vi "OS Simulator - V3.vi"() -> ()   [LabVIEW 2020]
uses:
  <vilib>/numeric/Random Number (Range) U64.vi
  <vilib>/numeric/Random Number (Range) DBL.vi
  <vilib>/numeric/Random Number (Range) I64.vi
  <vilib>/numeric/sub_Random U32.vi
panel:
  out "number":u64
  in  "Probabilidad de Memoria":dbl(slide)=15.0 min=0.0 max=80.0 step=1.0 scale=0.0..100.0
  in  "Numeric 4":dbl
  in  "Tamaño de Páginas":dbl(slide)=8.0 min=0.0 max=64.0 step=4.0 scale=4.0..64.0
  in  "Tamaño de Ram":dbl(slide)=64.0 min=0.0 max=80.0 step=4.0 scale=32.0..256.0
  in  "MEMORY MAP":string[](array[string])
  in  "TAP":string[][](table)
  in  "USING DISK":string
  in  "DISK WAITING":string[](array[string])
  in  "PROCESOS":dbl=20.0
  in  "VELOCIDAD":dbl(slide)=1000.0 min=0.0 max=2000.0 step=500.0
  in  "String":string
  in  "NEW":string[](array[string])
  in  "Numeric":dbl
  in  "FINISHED":string[](array[string])
  in  "PRINT":string
  in  "I/O WAITING":string[](array[string])
  in  "TABLA DE SALIDA":string[][](table)
  in  "RUNNING":string
  in  "READY":string[](array[string])
  in  "PROGRAM CONTROL BLOCK":string[][](table)
  in  "Tiempo Prom de Impresión":dbl(slide)=15.0 min=0.0 max=80.0 step=1.0 scale=10.0..80.0
  in  "Probabilidad de Impresión":dbl(slide)=50.0 min=0.0 max=100.0 step=1.0 scale=0.0..100.0
  in  "Duración Media de un Proceso":dbl(slide)=15.0 min=0.0 max=100.0 step=1.0 scale=0.0..100.0
  in  "Probabilidad de Proceso":dbl(slide) min=0.0 max=100.0 step=1.0 scale=0.0..100.0
  in  "Quantum":dbl(slide)=5.0 min=0.0 max=20.0 step=1.0 scale=0.0..20.0
  out "Play":bool
  out "Pause":bool
  in  "Play / Pause":bool=TRUE
  out "CLOCK":i32
  in  "Stop":bool
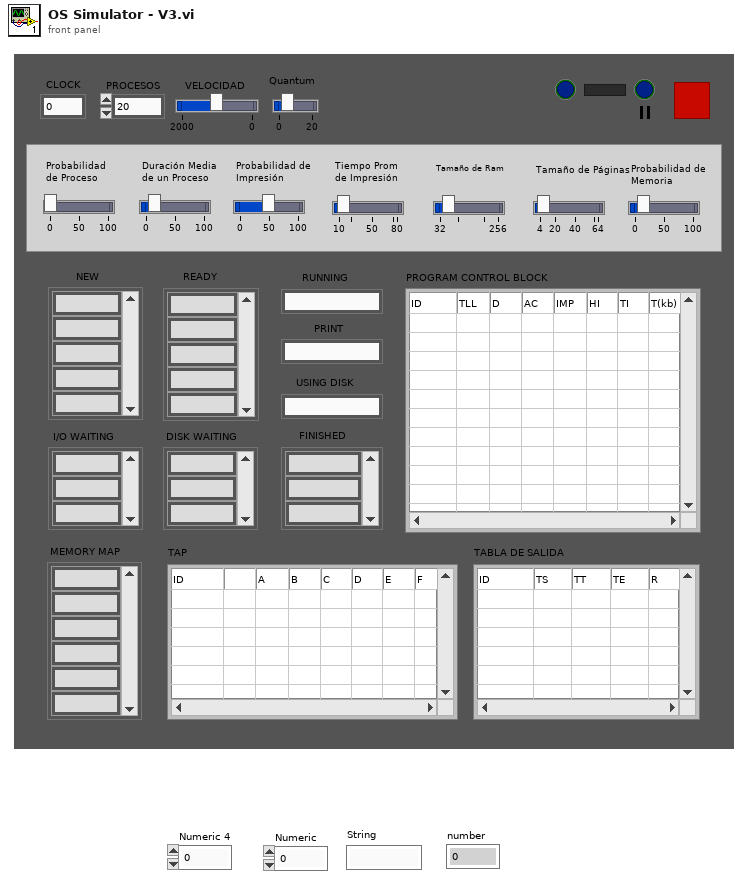
[diagram p1: front panel]
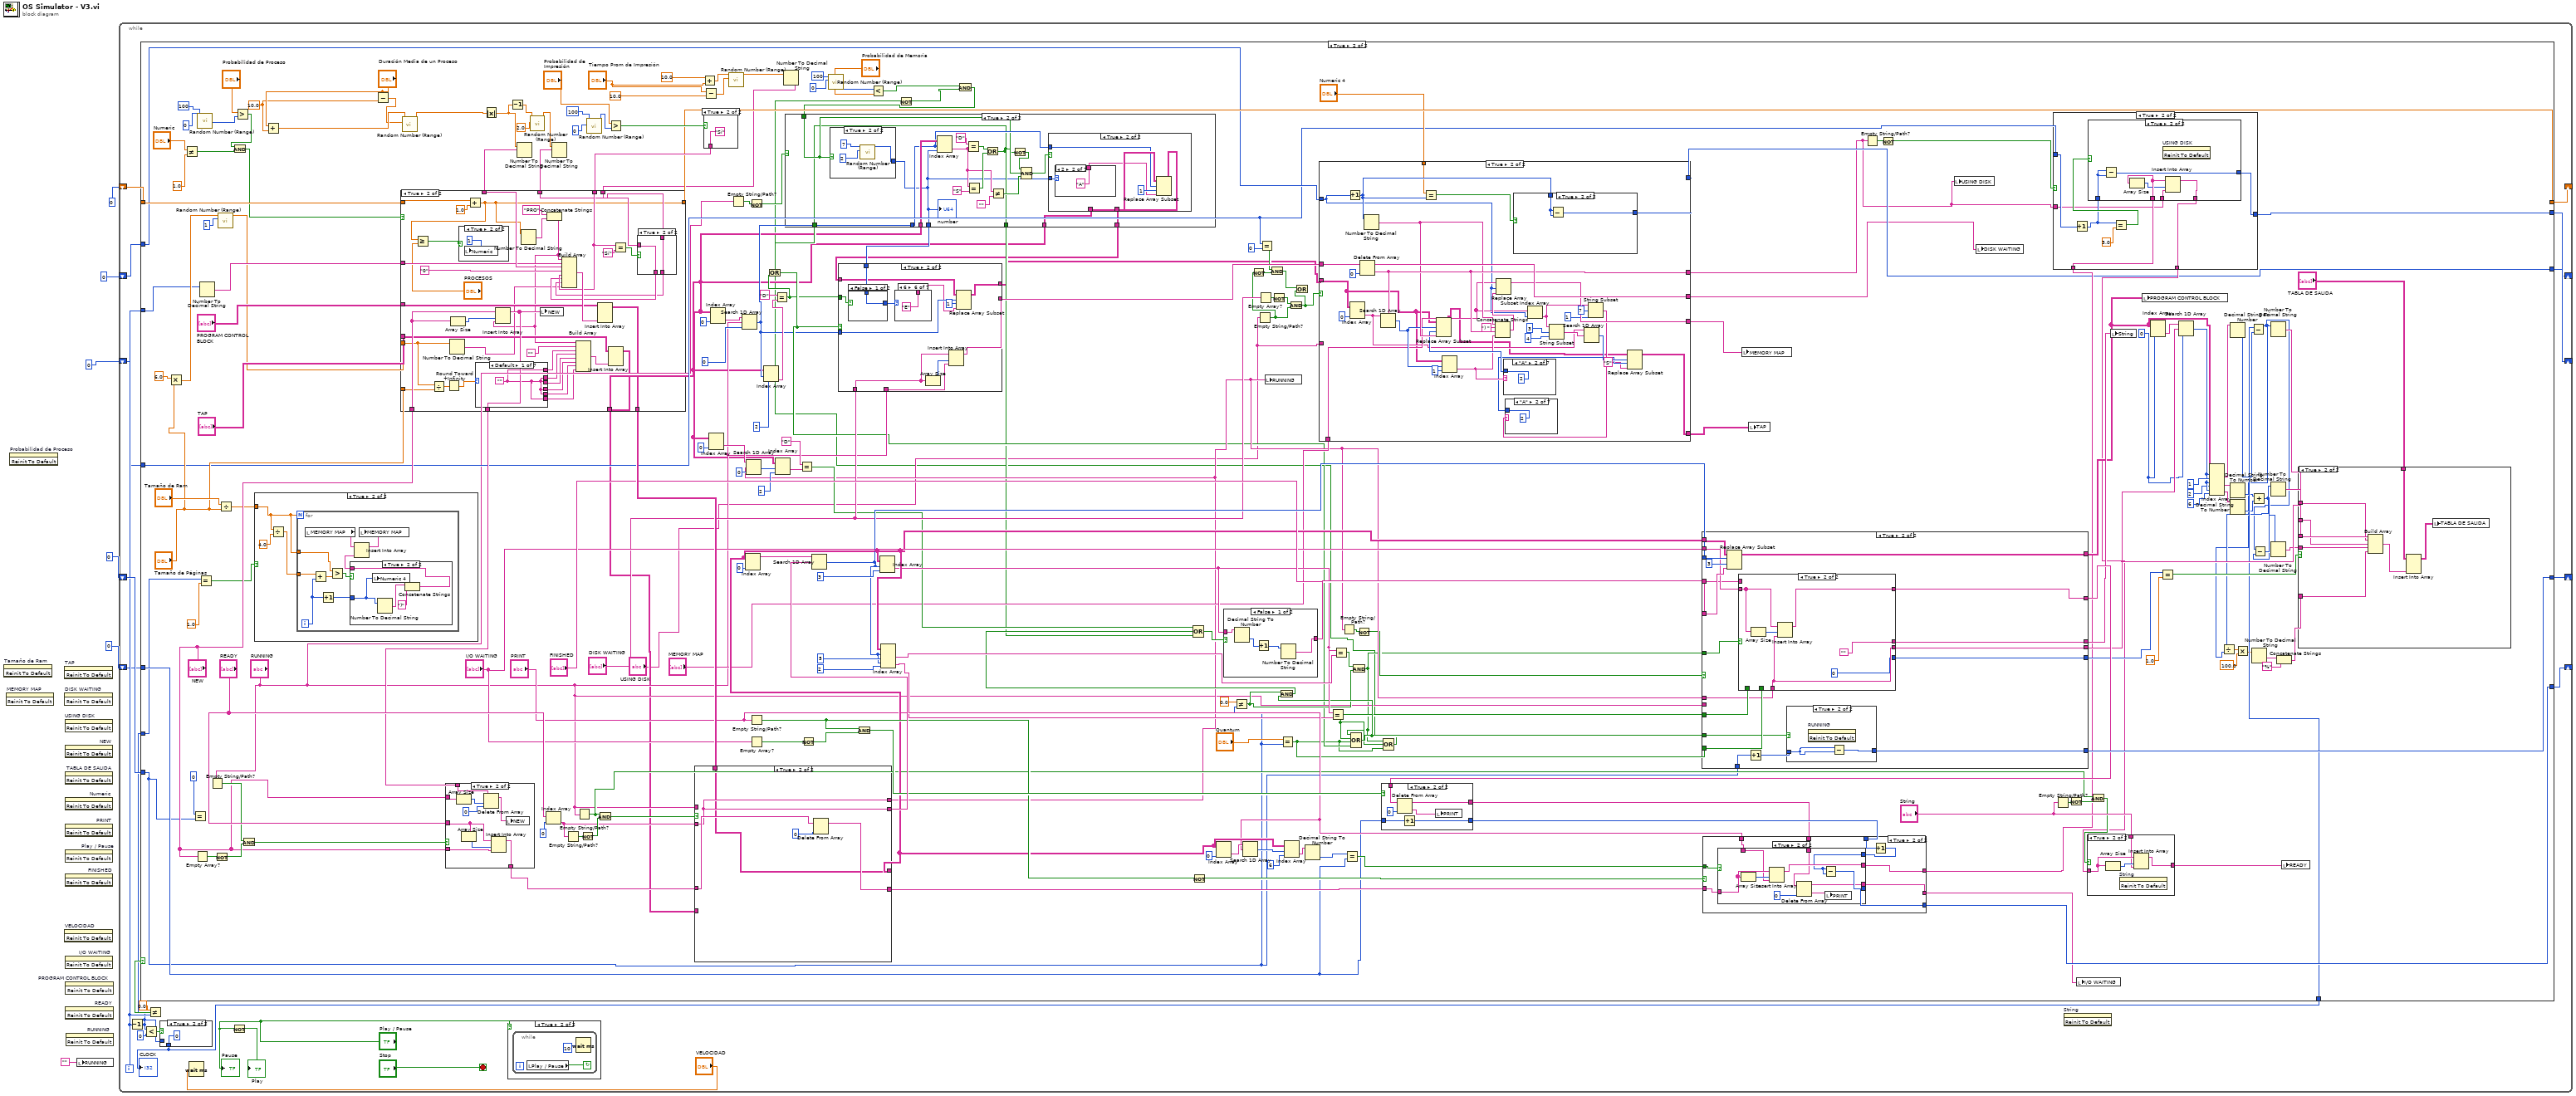
[diagram p0: block diagram]
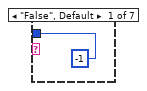
[diagram p5: hidden frame]
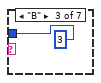
[diagram p6: hidden frame]
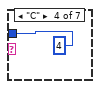
[diagram p7: hidden frame]
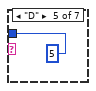
[diagram p8: hidden frame]
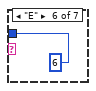
[diagram p9: hidden frame]
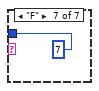
[diagram p10: hidden frame]
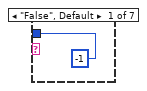
[diagram p11: hidden frame]
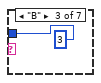
[diagram p12: hidden frame]
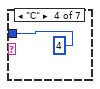
[diagram p13: hidden frame]
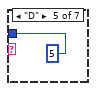
[diagram p14: hidden frame]
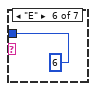
[diagram p15: hidden frame]
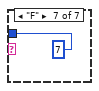
[diagram p16: hidden frame]
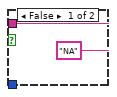
[diagram p19: hidden frame]
diagram:
  n1 = invoke on="Tamaño de Ram" class="Slide (strict)" method="Reinit To Default"() -> ()  [unwired: 3 in, 3 out]
  n2 = invoke on="MEMORY MAP" class="Arr (strict)" method="Reinit To Default"() -> ()  [unwired: 3 in, 3 out]
  n3 = invoke on="Probabilidad de Proceso" class="Slide (strict)" method="Reinit To Default"() -> ()  [unwired: 3 in, 3 out]
  n4 = invoke on="TAP" class="Tbl (strict)" method="Reinit To Default"() -> ()  [unwired: 3 in, 3 out]
  n5 = invoke on="DISK WAITING" class="Arr (strict)" method="Reinit To Default"() -> ()  [unwired: 3 in, 3 out]
  n6 = invoke on="VELOCIDAD" class="Slide (strict)" method="Reinit To Default"() -> ()  [unwired: 3 in, 3 out]
  n7 = invoke on="USING DISK" class="Str" method="Reinit To Default"() -> ()  [unwired: 3 in, 3 out]
  n8 = invoke on="NEW" class="Arr (strict)" method="Reinit To Default"() -> ()  [unwired: 3 in, 3 out]
  n9 = invoke on="TABLA DE SALIDA" class="Tbl (strict)" method="Reinit To Default"() -> ()  [unwired: 3 in, 3 out]
  n10 = invoke on="Numeric" class="DigNum (strict)" method="Reinit To Default"() -> ()  [unwired: 3 in, 3 out]
  n11 = invoke on="PRINT" class="Str" method="Reinit To Default"() -> ()  [unwired: 3 in, 3 out]
  n12 = invoke on="Play / Pause" class="Bool (strict)" method="Reinit To Default"() -> ()  [unwired: 3 in, 3 out]
  n13 = invoke on="FINISHED" class="Arr (strict)" method="Reinit To Default"() -> ()  [unwired: 3 in, 3 out]
  n14 = invoke on="I/O WAITING" class="Arr (strict)" method="Reinit To Default"() -> ()  [unwired: 3 in, 3 out]
  n15 = invoke on="PROGRAM CONTROL BLOCK" class="Tbl (strict)" method="Reinit To Default"() -> ()  [unwired: 3 in, 3 out]
  n16 = invoke on="READY" class="Arr (strict)" method="Reinit To Default"() -> ()  [unwired: 3 in, 3 out]
  n17 = invoke on="RUNNING" class="Str" method="Reinit To Default"() -> ()  [unwired: 3 in, 3 out]
  n18 = local write "RUNNING"("") -> ()
  n19 = while {
    shift-right: [w24] -> _
    shift-left: 0 -> [w23]
    shift-right: [w19] -> _
    shift-left: 0 -> [w20]
    shift-right: [w14] -> _
    shift-left: 0 -> [w15]
    shift-right: [w9] -> _
    shift-left: 0 -> [w10]
    shift-right: [w7] -> _
    shift-left: 0 -> [w8]
    i -> [w18]
    stop <- "Stop" stop-if-true
    n20 = Decrement(x=w18) -> (x-1=w11:i32)
    n21 = Less?(x=w11, y=0) -> (x < y?=w17:bool)
    n22 = Not Equal?(x=0.0, y=w18) -> (x != y?=w22:bool)
    n23 = case shown="True" w17 {
      tunnel: [w28 0] -> w13
      tunnel: w11 -> [w28 _]
      frame False {
      }
      frame True {
      }
    }
    "CLOCK" <- w13
    n24 = case shown="True" w22 {
      tunnel: [w34 w225] -> w24
      tunnel: w23 -> [w34 w224]
      tunnel: w18 -> [_ w113]
      tunnel: w20 -> [w33 w94]
      tunnel: [w33 w189] -> w19
      tunnel: w15 -> [w32 w168]
      tunnel: [w32 w178] -> w14
      tunnel: w13 -> [_ w142]
      tunnel: w11 -> [_ w110]
      tunnel: w10 -> [w31 w68]
      tunnel: [w31 w77] -> w9
      tunnel: w8 -> [w30 w74]
      tunnel: [w30 w73] -> w7
      frame False {
      }
      frame True {
        w130 = 0 ("disabled index (col)")
        w228 = 10.0 ("y")
        n25 = Multiply(x=6.0, y="Tamaño de Páginas") -> (x*y=w116:dbl)
        n26 = Not Equal?(x="Numeric", y=1.0) -> (x != y?=w210:bool)
        n27 = Equal?(x=0, y=w94) -> ()  [unwired: 1 out]
        n28 = Empty Array?(array="NEW") -> (empty?=w207:bool)
        n29 = call-poly <vilib>:"Random Number (Range).vi"("lower bound (-100)"=0, "upper bound (100)"=100) -> ("number"=w204:i64)  [unwired: 9 in]
        n30 = Equal?(x=w110, y=1.0) -> (x = y?=w112:bool)
        n31 = Number To Decimal String(number=w113) -> (decimal integer string=w237:string)  [unwired: 1 in]
        n32 = Empty String/Path?(string/path="RUNNING") -> (empty?=w200:bool)
        n33 = Not(x=w207) -> (.not. x?=w206:bool)
        n34 = call-poly <vilib>:"Random Number (Range).vi"("lower bound (0)"=1, "upper bound (100)"=w116) -> ("number"=w119:dbl)  [unwired: 9 in]
        n35 = Divide(x="Tamaño de Ram", y="Tamaño de Páginas") -> (x/y=w111:dbl)
        n36 = Greater?(x="Probabilidad de Proceso", y=w204) -> (0:w211:bool)
        n37 = And(x=w211, y=w210) -> (x .and. y?=w209:bool)
        n38 = And(x=w200, y=w206) -> (x .and. y?=w187:bool)
        n39 = case shown="True" w112 {
          tunnel: w111 -> [_ w300]
          frame False {
          }
          frame True {
            n40 = Divide(x=w300, y=4.0) -> (x/y=w301:dbl)
            n41 = for {
              N: w300 -> [_]
              tunnel: w301 -> [w309]
              tunnel: w300 -> [w306]
              i -> [w303]
              n42 = local read "MEMORY MAP"() -> (w310:string[])
              n43 = Add(x=w309, y=w303) -> (x+y=w305:dbl)
              n44 = Increment(x=w303) -> (x+1=w304:i32)
              n45 = Greater?(x=w306, y=w305) -> (0:w307:bool)
              n46 = case shown="True" w307 {
                tunnel: ["NA" w314] -> w308
                tunnel: w304 -> [_ w313]
                frame False {
                }
                frame True {
                  n47 = local write "Numeric 4"(w313) -> ()
                  n48 = Number To Decimal String(number=w313) -> (decimal integer string=w316:string)  [unwired: 1 in]
                  n49 = Concatenate Strings(w316, ")" ("string")) -> (w314:string)
                }
              }
              n50 = Insert Into Array(array=w310, new element=w308) -> (w311:string[])  [unwired: 1 in]
              n51 = local write "MEMORY MAP"(w311) -> ()
            }
          }
        }
        n52 = Add(x="Duración Media de un Proceso", y=w228) -> (x+y=w235:dbl)
        n53 = Subtract(x="Duración Media de un Proceso", y=w228) -> (x-y=w233:dbl)
        n54 = call-poly <vilib>:"Random Number (Range).vi"("lower bound (0)"=w233, "upper bound (100)"=w235) -> ("number"=w157:dbl)  [unwired: 9 in]
        n55 = Absolute Value(x=w157) -> (abs(x)=w156:dbl)
        n56 = Decrement(x=w156) -> (x-1=w216:dbl)
        n57 = Number To Decimal String(number=w156) -> (decimal integer string=w236:string)  [unwired: 1 in]
        n58 = call-poly <vilib>:"Random Number (Range).vi"("lower bound (0)"=2.0, "upper bound (100)"=w216) -> ("number"=w240:dbl)  [unwired: 9 in]
        n59 = Index Array(array="READY", index=0) -> (element=w242:string)
        n60 = Number To Decimal String(number=w240) -> (decimal integer string=w241:string)  [unwired: 1 in]
        n61 = Empty String/Path?(string/path=w242) -> (empty?=w243:bool)
        n62 = Empty String/Path?(string/path="RUNNING") -> (empty?=w159:bool)
        n63 = Not(x=w243) -> (.not. x?=w244:bool)
        n64 = call-poly <vilib>:"Random Number (Range).vi"("lower bound (-100)"=0, "upper bound (100)"=100) -> ("number"=w201:i64)  [unwired: 9 in]
        n65 = And(x=w159, y=w244) -> (x .and. y?=w158:bool)
        n66 = Greater?(x="Probabilidad de Impresión", y=w201) -> (0:w238:bool)
        n67 = Add(x=10.0, y="Tiempo Prom de Impresión") -> (x+y=w220:dbl)
        n68 = Subtract(x="Tiempo Prom de Impresión", y=10.0) -> (x-y=w219:dbl)
        n69 = case shown="True" w238 {
          tunnel: ["No" "Sí"] -> w239
          frame False {
          }
          frame True {
          }
        }
        n70 = call-poly <vilib>:"Random Number (Range).vi"("lower bound (0)"=w219, "upper bound (100)"=w220) -> ("number"=w218:dbl)  [unwired: 9 in]
        n71 = Empty String/Path?(string/path="RUNNING") -> (empty?=w57:bool)
        n72 = Not(x=w57) -> (.not. x?=w56:bool)
        n73 = Empty String/Path?(string/path="PRINT") -> (empty?=w180:bool)
        n74 = Empty Array?(array="I/O WAITING") -> (empty?=w185:bool)
        n75 = Number To Decimal String(number=w218) -> (decimal integer string=w217:string)  [unwired: 1 in]
        n76 = case shown="True" w209 {
          tunnel: "PROGRAM CONTROL BLOCK" -> [w522 w560]
          tunnel: w236 -> [_ w559]
          tunnel: w237 -> [_ w558]
          tunnel: w239 -> [_ w553]
          tunnel: w241 -> [_ w550]
          tunnel: w224 -> [w523 w554]
          tunnel: [w523 w544] -> w225
          tunnel: w217 -> [_ w547]
          tunnel: [w522 w548] -> w214
          tunnel: "NEW" -> [w521 w543]
          tunnel: [w521 w541] -> w198
          tunnel: "TAP" -> [w520 w538]
          tunnel: [w520 w537] -> w45
          tunnel: w119 -> [_ w536]
          tunnel: "Tamaño de Páginas" -> [_ w535]
          frame False {
          }
          frame True {
            n77 = Divide(x=w536, y=w535) -> (x/y=w534:dbl)
            n78 = Round Toward +Infinity(x=w534) -> (ceil(x): smallest int >= x=w533:dbl)
            n79 = Number To Decimal String(number=w536) -> (decimal integer string=w526:string)  [unwired: 1 in]
            n80 = Array Size(array=w543) -> (size(s)=w542:i32)
            n81 = Add(x=w554, y=1.0) -> (x+y=w544:dbl)
            n82 = Greater Or Equal?(x=w544, y="PROCESOS") -> (x >= y?=w545:bool)
            n83 = case shown="True" w545 {
              frame False {
              }
              frame True {
                n84 = local write "Numeric"(1) -> ()
              }
            }
            n85 = case shown="Default" w533 {
              tunnel: [w563 "D" w567 w568 w571 w572 w574] -> w532
              tunnel: [w563 w564 w567 w568 w571 w572 w574] -> w531
              tunnel: [w563 w564 w566 w568 w571 w572 w574] -> w530
              tunnel: [w563 w564 w566 w569 w571 w572 w574] -> w529
              tunnel: [w563 w564 w566 w569 w570 w572 w574] -> w528
              tunnel: [w563 w564 w566 w569 w570 "" w574] -> w527
              frame Default {
                w563 = ""
              }
              frame 1 {
                w564 = ""
              }
              frame 2 {
                w566 = ""
                w567 = "D"
              }
              frame 3 {
                w568 = "D"
                w569 = ""
              }
              frame 4 {
                w570 = ""
                w571 = "D"
              }
              frame 5 {
                w572 = "D"
              }
              frame 6 {
                w574 = "D"
              }
            }
            n86 = Number To Decimal String(number=w544) -> (decimal integer string=w556:string)  [unwired: 1 in]
            n87 = Concatenate Strings("PRO", w556) -> (w525:string)
            n88 = Insert Into Array(array=w543, index=w542, new element=w525) -> (w541:string[])
            n89 = local write "NEW"(w541) -> ()
            n90 = Build Array(w525, "", w532, w531, w530, w529, w528, w527) -> (w539:string[])
            n91 = Insert Into Array(array=w538, new element=w539) -> (w537:string[][])  [unwired: 2 in]
            n92 = Equal?(x=w553, y="Sí") -> (x = y?=w551:bool)
            n93 = case shown="True" w551 {
              tunnel: w550 -> [_ w578]
              tunnel: [w576 w578] -> w549
              tunnel: [w576 w577] -> w546
              tunnel: w547 -> [_ w577]
              frame False {
                w576 = ""
              }
              frame True {
              }
            }
            n94 = Build Array(w525, w558, w559, "0", w553, w549, w546, w526) -> (w562:string[])
            n95 = Insert Into Array(array=w560, new element=w562) -> (w548:string[][])  [unwired: 2 in]
          }
        }
        n96 = case shown="True" w187 {
          tunnel: "READY" -> [w430 w439]
          tunnel: [w430 w431] -> w188
          tunnel: "NEW" -> [_ w437]
          tunnel: "NEW" -> [_ w432]
          tunnel: w198 -> [_ w434]
          frame False {
          }
          frame True {
            n97 = Array Size(array=w432) -> (size(s)=w433:i32)
            n98 = Array Size(array=w439) -> (size(s)=w438:i32)
            n99 = Delete From Array(array=w434, length=w433, index=0) -> (array with subset deleted=w436:string[])  [unwired: 1 out]
            n100 = Insert Into Array(array=w439, index=w438, new element=w437) -> (w431:string[])
            n101 = local write "NEW"(w436) -> ()
          }
        }
        n102 = case shown="True" w158 {
          tunnel: w242 -> [_ w426]
          tunnel: w188 -> [w424 w429]
          tunnel: [w424 w428] -> w171
          tunnel: w214 -> [w423 w425]
          tunnel: [w423 w425] -> w175
          tunnel: [w422 w426] -> w186
          tunnel: "RUNNING" -> [w422 _]
          tunnel: w45 -> [_ _]
          tunnel: [w422 w426] -> w70
          frame False {
          }
          frame True {
            n103 = Delete From Array(array=w429, index=0) -> (array with subset deleted=w428:string[])  [unwired: 1 in, 1 out]
          }
        }
        n104 = Index Array(array=w45, index (col)=0 ("disabled index (col)")) -> (element=w90:string[])  [unwired: 1 in]
        n105 = Index Array(array=w45, index (col)=0 ("disabled index (col)")) -> (element=w108:string[])  [unwired: 1 in]
        n106 = Search 1D Array(1D array=w108, element="RUNNING", start index (0)=0) -> (index of element=w51:i32)
        n107 = Index Array(array=w175, index (col)=0 ("disabled index (col)")) -> (element=w196:string[])  [unwired: 1 in]
        n108 = Search 1D Array(1D array=w90, element=w70, start index (0)=0) -> (index of element=w87:i32)
        n109 = Index Array(array=w45, index (row)=w51, index (col)=2 ("disabled index (col)")) -> (element=w105:string)
        n110 = Equal?(x="D", y=w105) -> (x = y?=w52:bool)
        n111 = Index Array(array=w45, index (row)=w87, index (col)=2) -> (element=w86:string)
        n112 = Equal?(x="D", y=w86) -> (x = y?=w84:bool)
        n113 = Not(x=w185) -> (.not. x?=w181:bool)
        n114 = Search 1D Array(1D array=w196, element=w186) -> (index of element=w193:i32)  [unwired: 1 in]
        n115 = call-poly <vilib>:"Random Number (Range).vi"("lower bound (0)"=u64 0, "upper bound (100)"=u64 100) -> ("number"=w60:u64)  [unwired: 9 in]
        n116 = And(x=w180, y=w181) -> (x .and. y?=w182:bool)
        n117 = Less?(x=w60, y="Probabilidad de Memoria") -> (x < y?=w49:bool)
        n118 = Index Array(array=w175, index (row)=w193, index (col)=3 ("disabled index (col)")) -> (element=w98:string)
        n119 = Index Array(array=w175, index (row) #1=w193, index (col) #1=5 ("disabled index (col)"), index (row) #2=w193, index (col) #2=2 ("disabled index (col)")) -> (element #1=w161:string, element #2=w160:string)
        n120 = Not(x=w180) -> (.not. x?=w179:bool)
        n121 = Index Array(array=w175, index (col)=0 ("disabled index (col)")) -> (element=w177:string[])  [unwired: 1 in]
        n122 = Not Equal?(x=0.0, y=w94) -> (x != y?=w93:bool)
        n123 = Search 1D Array(1D array=w177, element="PRINT") -> (index of element=w174:i32)  [unwired: 1 in]
        n124 = Empty String/Path?(string/path="USING DISK") -> (empty?=w66:bool)
        n125 = Not(x=w66) -> (.not. x?=w65:bool)
        n126 = Empty Array?(array="DISK WAITING") -> (empty?=w103:bool)
        n127 = Equal?(x=w68, y=0) -> (x = y?=w64:bool)
        n128 = local write "RUNNING"(w70) -> ()
        n129 = And(x=w64, y=w65) -> (x .and. y?=w63:bool)
        n130 = Not(x=w103) -> (.not. x?=w102:bool)
        n131 = Equal?(x="Quantum", y=w94) -> (x = y?=w38:bool)
        n132 = Index Array(array=w175, index (row)=w174, index (col)=6 ("disabled index (col)")) -> (element=w169:string)
        n133 = And(x=w102, y=w66) -> (x .and. y?=w62:bool)
        n134 = Or(x=w63, y=w62) -> ()  [unwired: 1 out]
        n135 = Decimal String To Number(string=w169) -> (number=w92:i32)  [unwired: 2 in, 1 out]
        n136 = Equal?(x=w98, y=w160) -> (x = y?=w37:bool)
        n137 = Equal?(x=w98, y=w161) -> (x = y?=w42:bool)
        n138 = Empty String/Path?(string/path=w70) -> (empty?=w99:bool)
        n139 = Equal?(x=w92, y=w168) -> (x = y?=w172:bool)
        n140 = And(x=w42, y=w93) -> (x .and. y?=w36:bool)
        n141 = Not(x=w99) -> (.not. x?=w69:bool)
        n142 = Compound Arithmetic op=OR(w36, w37, w38) -> (w35:bool)
        n143 = Not(x=w35) -> (.not. x?=w50:bool)
        n144 = And(x=w49, y=w50) -> (x .and. y?=w48:bool)
        n145 = case shown="True" w56 {
          tunnel: w48 -> [_ w450]
          tunnel: [w441 w444] -> w54
          tunnel: w45 -> [_ w458]
          tunnel: w51 -> [_ w452]
          tunnel: w45 -> [w442 w453]
          tunnel: [w442 w451] -> w44
          tunnel: [w441 w444] -> w47
          tunnel: [-1 w443] -> w46
          frame False {
            w441 = FALSE
          }
          frame True {
            n146 = case shown="True" w450 {
              tunnel: [0 w474] -> w443
              frame False {
              }
              frame True {
                n147 = call-poly <vilib>:"Random Number (Range).vi"("lower bound (0)"=u64 2, "upper bound (100)"=u64 7) -> ("number"=w474:u64)  [unwired: 9 in]
              }
            }
            "number" <- w443
            n148 = Index Array(array=w458, index (row)=w452, index (col)=w443) -> (element=w447:string)
            n149 = Equal?(x="D", y=w447) -> (x = y?=w456:bool)
            n150 = Equal?(x=w447, y="S") -> (x = y?=w455:bool)
            n151 = Or(x=w456, y=w455) -> (x .or. y?=w444:bool)
            n152 = Not Equal?(x=w447, y="") -> (x != y?=w445:bool)
            n153 = Not(x=w444) -> (.not. x?=w449:bool)
            n154 = Compound Arithmetic op=AND(w449, w450, w445) -> (w448:bool)
            n155 = case shown="True" w448 {
              tunnel: w453 -> [w459 w465]
              tunnel: w452 -> [_ w464]
              tunnel: [w459 w462] -> w451
              tunnel: w443 -> [_ w461]
              frame False {
              }
              frame True {
                n156 = case shown="2" w461 {
                  tunnel: ["" "A" "B" "C" "D" "E" "F"] -> w460
                  frame 0, Default {
                  }
                  frame 2 {
                  }
                  frame 3 {
                  }
                  frame 4 {
                  }
                  frame 5 {
                  }
                  frame 6 {
                  }
                  frame 7 {
                  }
                }
                n157 = Replace Array Subset(array=w465, new element=w460, index (row)=w464, index (col)=1 ("disabled index (col)")) -> (w462:string[][])
              }
            }
          }
        }
        n158 = Or(x=w54, y=w52) -> (x .or. y?=w53:bool)
        n159 = case shown="True" w53 {
          tunnel: "DISK WAITING" -> [w496 w507]
          tunnel: "RUNNING" -> [_ w508]
          tunnel: [w496 w505] -> w100
          tunnel: w52 -> [_ w504]
          tunnel: w51 -> [_ w500]
          tunnel: w46 -> [_ w502]
          tunnel: w44 -> [w495 w501]
          tunnel: [w495 w497] -> w43
          frame False {
          }
          frame True {
            n160 = case shown="False" w504 {
              tunnel: [w509 2] -> w503
              tunnel: w502 -> [w509 _]
              frame False {
              }
              frame True {
              }
            }
            n161 = case shown="6" w503 {
              tunnel: ["" "A" "B" "C" "D" "E" "F"] -> w498
              frame 0, Default {
              }
              frame 2 {
              }
              frame 3 {
              }
              frame 4 {
              }
              frame 5 {
              }
              frame 6 {
              }
              frame 7 {
              }
            }
            n162 = Array Size(array=w507) -> (size(s)=w506:i32)
            n163 = Insert Into Array(array=w507, index=w506, new element=w508) -> (w505:string[])
            n164 = Replace Array Subset(array=w501, new element=w498, index (row)=w500, index (col)=1 ("disabled index (col)")) -> (w497:string[][])
          }
        }
        n165 = case shown="True" w62 {
          tunnel: w100 -> [w249 w281]
          tunnel: [w249 w279] -> w40
          tunnel: w43 -> [w248 w259]
          tunnel: [w248 w250] -> w81
          tunnel: "MEMORY MAP" -> [w245 w265]
          tunnel: [w247 w278] -> w39
          tunnel: "USING DISK" -> [w247 _]
          tunnel: w74 -> [w246 w264]
          tunnel: [w246 w271] -> w73
          tunnel: [w245 w274] -> w72
          tunnel: "Numeric 4" -> [_ w270]
          frame False {
          }
          frame True {
            n166 = Increment(x=w264) -> (x+1=w272:i32)
            n167 = Index Array(array=w259, index (col)=0 ("disabled index (col)")) -> (element=w260:string[])  [unwired: 1 in]
            n168 = Delete From Array(array=w281, index=0) -> (deleted portion=w278:string, array with subset deleted=w279:string[])  [unwired: 1 in]
            n169 = Number To Decimal String(number=w272) -> (decimal integer string=w275:string)  [unwired: 1 in]
            n170 = Search 1D Array(1D array=w260, element=w278) -> (index of element=w268:i32)  [unwired: 1 in]
            n171 = Equal?(x=w270, y=w272) -> (x = y?=w273:bool)
            n172 = Index Array(array=w259, index (row)=w268, index (col)=1 ("disabled index (col)")) -> (element=w266:string)
            n173 = Concatenate Strings(w275, ") " ("string"), w278, w266) -> (w277:string)
            n174 = Replace Array Subset(array=w265, new element=w277, index=w264) -> (w274:string[])
            n175 = case shown="\"A\"" w266 {
              tunnel: [-1 2 3 4 5 6 7] -> w267
              frame "False", Default {
              }
              frame "A" {
              }
              frame "B" {
              }
              frame "C" {
              }
              frame "D" {
              }
              frame "E" {
              }
              frame "F" {
              }
            }
            n176 = Replace Array Subset(array=w259, new element=w275, index (row)=w268, index (col)=w267) -> (w251:string[][])
            n177 = case shown="True" w273 {
              tunnel: w272 -> [w297 w299]
              tunnel: [w297 w298] -> w271
              frame False {
              }
              frame True {
                n178 = Subtract(x=w299, y=w299) -> (x-y=w298:i32)
              }
            }
            n179 = Index Array(array=w265, index=w264) -> (element=w257:string)
            n180 = String Subset(string=w257, offset (0)=3, length (rest)=4 ("length (rest)")) -> (substring=w261:string)
            n181 = Search 1D Array(1D array=w260, element=w261) -> (index of element=w258:i32)  [unwired: 1 in]
            n182 = String Subset(string=w257, offset (0)=7, length (rest)=1 ("length (rest)")) -> (substring=w254:string)
            n183 = case shown="\"A\"" w254 {
              tunnel: [-1 2 3 4 5 6 7] -> w253
              frame "False", Default {
              }
              frame "A" {
              }
              frame "B" {
              }
              frame "C" {
              }
              frame "D" {
              }
              frame "E" {
              }
              frame "F" {
              }
            }
            n184 = Replace Array Subset(array=w251, new element="S" ("new element/subarray"), index (row)=w258, index (col)=w253) -> (w250:string[][])
          }
        }
        n185 = Compound Arithmetic op=OR(w36, w37, w38, w53) -> (w95:bool)
        n186 = And(x=w93, y=w95) -> (x .and. y?=w83:bool)
        n187 = Compound Arithmetic op=OR(w84, w83, w47) -> (w82:bool)
        n188 = case shown="False" w82 {
          tunnel: w98 -> [w418 w421]
          tunnel: [w417 w421] -> w191
          frame False {
            n189 = Decimal String To Number(string=w418) -> (number=w420:i32)  [unwired: 2 in, 1 out]
            n190 = Increment(x=w420) -> (x+1=w419:i32)
            n191 = Number To Decimal String(number=w419) -> (decimal integer string=w417:string)  [unwired: 1 in]
          }
          frame True {
          }
        }
        n192 = case shown="True" w69 {
          tunnel: w175 -> [w368 w387]
          tunnel: w193 -> [_ w386]
          tunnel: w191 -> [_ w384]
          tunnel: [w368 w383] -> w151
          tunnel: w36 -> [_ w375]
          tunnel: "RUNNING" -> [w364 _]
          tunnel: "I/O WAITING" -> [w367 w382]
          tunnel: [w367 w381] -> w184
          tunnel: w37 -> [_ w374]
          tunnel: "FINISHED" -> [_ w380]
          tunnel: w94 -> [w366 w378]
          tunnel: [w366 w379] -> w189
          tunnel: w38 -> [_ w376]
          tunnel: ["" w373] -> w152
          tunnel: [w364 w372] -> w146
          tunnel: [0 w371] -> w145
          tunnel: w70 -> [_ w370]
          tunnel: w95 -> [_ w369]
          frame False {
          }
          frame True {
            n193 = Replace Array Subset(array=w387, new element=w384, index (row)=w386, index (col)=3 ("disabled index (col)")) -> (w383:string[][])
            n194 = case shown="True" w375 {
              tunnel: w370 -> [w396 w412]
              tunnel: w382 -> [w398 w415]
              tunnel: [w398 w414] -> w381
              tunnel: w374 -> [w397 _]
              tunnel: w380 -> [w395 _]
              tunnel: w376 -> [w394 _]
              tunnel: [w393 ""] -> w373
              tunnel: [w392 w412] -> w372
              tunnel: [w391 0] -> w371
              frame False {
                n195 = case shown="True" w397 {
                  tunnel: w396 -> [w400 w406]
                  tunnel: w395 -> [_ w409]
                  tunnel: w394 -> [w402 _]
                  tunnel: [w401 ""] -> w393
                  tunnel: [w400 w406] -> w392
                  tunnel: [0 1] -> w391
                  frame False {
                    n196 = case shown="True" w402 {
                      tunnel: w400 -> [_ w404]
                      tunnel: ["" w404] -> w401
                      frame False {
                      }
                      frame True {
                      }
                    }
                  }
                  frame True {
                    n197 = Array Size(array=w409) -> (size(s)=w410:i32)
                    n198 = Insert Into Array(array=w409, index=w410, new element=w406) -> (w407:string[])
                    n199 = local write "FINISHED"(w407) -> ()
                  }
                }
              }
              frame True {
                n200 = Array Size(array=w415) -> (size(s)=w416:i32)
                n201 = Insert Into Array(array=w415, index=w416, new element=w412) -> (w414:string[])
              }
            }
            n202 = Increment(x=w378) -> (x+1=w377:i32)
            n203 = case shown="True" w369 {
              tunnel: w377 -> [w388 w390]
              tunnel: [w388 w389] -> w379
              frame False {
              }
              frame True {
                n204 = invoke on="RUNNING" class="Str" method="Reinit To Default"() -> ()  [unwired: 3 in, 3 out]
                n205 = Subtract(x=w390, y=w390) -> (x-y=w389:i32)
              }
            }
          }
        }
        n206 = case shown="True" w182 {
          tunnel: w184 -> [w356 w362]
          tunnel: [w356 w359] -> w148
          tunnel: w168 -> [w355 w358]
          tunnel: [w355 w357] -> w167
          frame False {
          }
          frame True {
            n207 = Delete From Array(array=w362, index=0) -> (deleted portion=w360:string, array with subset deleted=w359:string[])  [unwired: 1 in]
            n208 = Increment(x=w358) -> (x+1=w357:i32)
            n209 = local write "PRINT"(w360) -> ()
          }
        }
        n210 = case shown="True" w179 {
          tunnel: [w331 w335] -> w178
          tunnel: w172 -> [_ w341]
          tunnel: w171 -> [w332 w340]
          tunnel: "PRINT" -> [_ w339]
          tunnel: [w332 w338] -> w76
          tunnel: w167 -> [w331 w337]
          tunnel: w148 -> [w330 w334]
          tunnel: [w330 w333] -> w147
          frame False {
          }
          frame True {
            n211 = Increment(x=w337) -> (x+1=w336:i32)
            n212 = case shown="True" w341 {
              tunnel: w340 -> [w344 w354]
              tunnel: w339 -> [_ w352]
              tunnel: [w344 w351] -> w338
              tunnel: w336 -> [w343 w350]
              tunnel: [w343 w349] -> w335
              tunnel: w334 -> [w342 w348]
              tunnel: [w342 w345] -> w333
              frame False {
              }
              frame True {
                n213 = Array Size(array=w354) -> (size(s)=w353:i32)
                n214 = Insert Into Array(array=w354, index=w353, new element=w352) -> (w351:string[])
                n215 = Delete From Array(array=w348, index=0) -> (deleted portion=w346:string, array with subset deleted=w345:string[])  [unwired: 1 in]
                n216 = Subtract(x=w350, y=w350) -> (x-y=w349:i32)
                n217 = local write "PRINT"(w346) -> ()
              }
            }
          }
        }
        n218 = local write "MEMORY MAP"(w72) -> ()
        n219 = local write "TAP"(w81) -> ()
        n220 = Empty String/Path?(string/path=w39) -> (empty?=w79:bool)
        n221 = Not(x=w79) -> (.not. x?=w78:bool)
        n222 = local write "USING DISK"(w39) -> ()
        n223 = local write "DISK WAITING"(w40) -> ()
        n224 = case shown="True" w78 {
          tunnel: w68 -> [w478 w486]
          tunnel: [w478 w482] -> w77
          tunnel: w76 -> [w477 w481]
          tunnel: [w477 w480] -> w75
          tunnel: w39 -> [_ w479]
          frame False {
          }
          frame True {
            n225 = Increment(x=w486) -> (x+1=w483:i32)
            n226 = Equal?(x=w483, y=3.0) -> (x = y?=w484:bool)
            n227 = case shown="True" w484 {
              tunnel: [w488 w494] -> w482
              tunnel: w483 -> [w488 w493]
              tunnel: w481 -> [w487 w492]
              tunnel: [w487 w490] -> w480
              tunnel: w479 -> [_ w489]
              frame False {
              }
              frame True {
                n228 = Subtract(x=w493, y=w493) -> (x-y=w494:i32)
                n229 = Array Size(array=w492) -> (size(s)=w491:i32)
                n230 = invoke on="USING DISK" class="Str" method="Reinit To Default"() -> ()  [unwired: 3 in, 3 out]
                n231 = Insert Into Array(array=w492, index=w491, new element=w489) -> (w490:string[])
              }
            }
          }
        }
        n232 = Empty String/Path?(string/path="String") -> (empty?=w164:bool)
        n233 = Not(x=w164) -> (.not. x?=w163:bool)
        n234 = local write "I/O WAITING"(w147) -> ()
        n235 = And(x=w159, y=w163) -> (x .and. y?=w162:bool)
        n236 = case shown="True" w162 {
          tunnel: w75 -> [w325 w329]
          tunnel: "String" -> [_ w327]
          tunnel: [w325 w326] -> w166
          frame False {
          }
          frame True {
            n237 = Array Size(array=w329) -> (size(s)=w328:i32)
            n238 = invoke on="String" class="Str" method="Reinit To Default"() -> ()  [unwired: 3 in, 3 out]
            n239 = Insert Into Array(array=w329, index=w328, new element=w327) -> (w326:string[])
          }
        }
        n240 = local write "String"(w152) -> ()
        n241 = local write "PROGRAM CONTROL BLOCK"(w151) -> ()
        n242 = Index Array(array=w151, index (col)=w130) -> (element=w153:string[])  [unwired: 1 in]
        n243 = Equal?(x=w145, y=1.0) -> (x = y?=w154:bool)
        n244 = Search 1D Array(1D array=w153, element=w146, start index (0)=w130) -> (index of element=w140:i32)
        n245 = Index Array(array=w151, index (row) #1=w140, index (col) #1=1 ("disabled index (col)"), index (row) #2=w140, index (col) #2=2 ("disabled index (col)"), index (row) #3=w140, index (col) #3=6 ("disabled index (col)")) -> (element #1=w144:string, element #2=w131:string, element #3=w132:string)
        n246 = Decimal String To Number(string=w144) -> (number=w143:i32)  [unwired: 2 in, 1 out]
        n247 = Decimal String To Number(string=w131) -> (number=w137:i32)  [unwired: 2 in, 1 out]
        n248 = Decimal String To Number(string=w132) -> (number=w136:i32)  [unwired: 2 in, 1 out]
        n249 = Subtract(x=w142, y=w143) -> (x-y=w128:i32)
        n250 = Add(x=w137, y=w136) -> (x+y=w129:i32)
        n251 = Divide(x=w129, y=w128) -> (x/y=w127:dbl)
        n252 = Multiply(x=w127, y=100.0) -> (x*y=w125:dbl)
        n253 = Number To Decimal String(number=w125) -> (decimal integer string=w124:string)  [unwired: 1 in]
        n254 = Subtract(x=w128, y=w129) -> (x-y=w134:i32)
        n255 = Number To Decimal String(number=w128) -> (decimal integer string=w141:string)  [unwired: 1 in]
        n256 = Number To Decimal String(number=w129) -> (decimal integer string=w135:string)  [unwired: 1 in]
        n257 = Number To Decimal String(number=w134) -> (decimal integer string=w133:string)  [unwired: 1 in]
        n258 = Concatenate Strings(w124, "%" ("string")) -> (w122:string)
        n259 = local write "READY"(w166) -> ()
        n260 = case shown="True" w154 {
          tunnel: "TABLA DE SALIDA" -> [_ w322]
          tunnel: w146 -> [_ w321]
          tunnel: w141 -> [_ w320]
          tunnel: w135 -> [_ w319]
          tunnel: w133 -> [_ w318]
          tunnel: w122 -> [_ w317]
          frame False {
          }
          frame True {
            n261 = Build Array(w321, w320, w319, w318, w317) -> (w323:string[])
            n262 = Insert Into Array(array=w322, new element=w323) -> (w324:string[][])  [unwired: 2 in]
            n263 = local write "TABLA DE SALIDA"(w324) -> ()
          }
        }
      }
    }
    n264 = Wait (ms)(milliseconds to wait="VELOCIDAD") -> ()  [unwired: 1 out]
    n265 = Not(x="Play / Pause") -> (.not. x?=→"Play":bool)
    n266 = case shown="True" "Play / Pause" {
      frame False {
      }
      frame True {
        n267 = while {
          stop <- w579 continue-if-true
          n268 = local read "Play / Pause"() -> (w579:bool)
          n269 = Wait (ms)(milliseconds to wait=u32 10) -> ()  [unwired: 1 out]
        }
      }
    }
    n270 = invoke on="String" class="Str" method="Reinit To Default"() -> ()  [unwired: 3 in, 3 out]
    "Pause" <- "Play / Pause"
  }
